vi "CreateListener.vi"(8 "error in (no error)":errorcluster, 11 "TCPIP in":refnum<class "TCPIP.lvclass">) -> (0 "error out":errorcluster, 3 "TCPIP out":refnum<class "TCPIP.lvclass">)   [LabVIEW 2018, in "TCPIP.lvclass"]
uses:
  TCPIP.lvclass
  TCPIP.lvclass/TCPIP.ctl
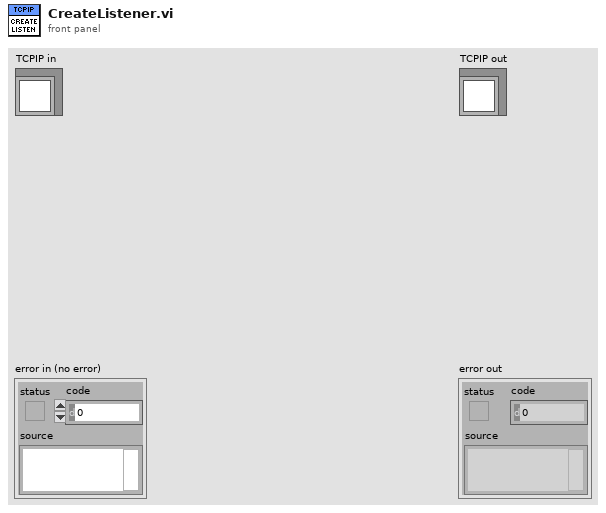
[diagram p1: front panel]
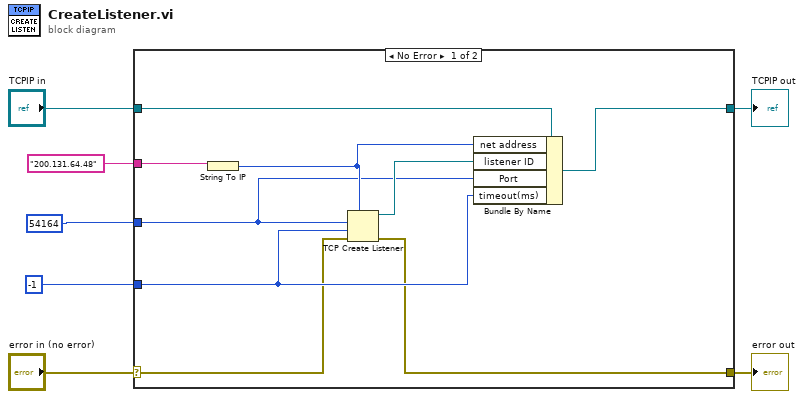
[diagram p0: block diagram]
diagram:
  n1 = case shown="No Error" "error in (no error)" {
    selector: "error in (no error)" -> [w9 w18]
    tunnel: [w8 w18] -> w6
    tunnel: [w15 w17] -> w4
    tunnel: "TCPIP in" -> [w16 w17]
    tunnel: "200.131.64.48" ("IP") -> [w14 _]
    tunnel: u16 54164 ("remote port") -> [w11 _]
    tunnel: -1 ("timeout") -> [w10 _]
    frame No Error {
      n2 = String To IP(1:w14) -> (0:w13:u32)
      n3 = TCP Create Listener(7:w13, 8:w9, 9:w10, 10:w11) -> (0:w8:errorcluster, 3:w12:refnum<k5>)  [unwired: 1 in, 1 out]
      n4 = Bundle By Name(cluster=w16, "net address"=w13, "listener ID"=w12, "Port"=w11, "timeout(ms)"=w10) -> (w15:refnum<class "TCPIP.lvclass">)
    }
    frame Error {
    }
  }
  "error out" <- w6
  "TCPIP out" <- w4
